vi "Init.vi"(8 "error in (no error)":errorcluster, 10 "Channel":i16, 11 "TrialBasedExperiment in":refnum<class "MouseMultiDim.lvclass">) -> (0 "error out":errorcluster, 3 "TrialBasedExperiment out":refnum<class "MouseMultiDim.lvclass">)   [LabVIEW 2014, in "MouseMultiDim.lvclass"]
uses:
  MouseMultiDim.lvclass
  Trial Based Experiment Statechart/PassiveExperiment/PassiveExperiment.lvclass
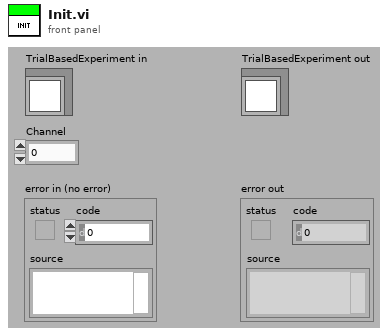
[diagram p1: front panel]
types:
  T1 = cluster{"Intertrial":dbl, "AcquireFixation":dbl, "HoldFixation":dbl, "DelayPeriod":dbl, "ResponsePeriod":dbl}
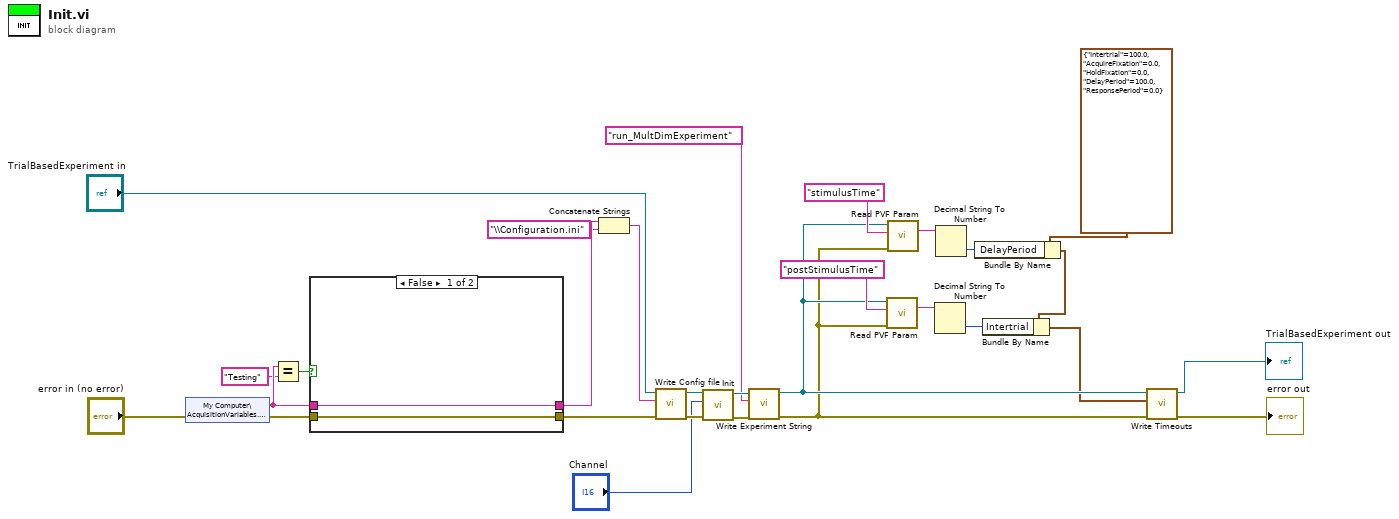
[diagram p0: block diagram]
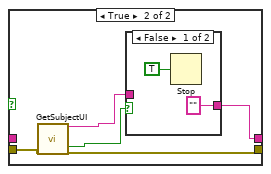
[diagram p2: hidden frame]
diagram:
  n1 = shared-variable "My Computer\\AcquisitionVariables.lvlib\\Subject"(error in="error in (no error)") -> (w26:string, error out=w27:errorcluster)
  n2 = Equal?(x=w26, y="Testing") -> (x = y?=w24:bool)
  n3 = case shown="False" w24 {
    tunnel: [w31 w36] -> w29
    tunnel: w26 -> [w31 _]
    tunnel: w27 -> [w30 w32]
    tunnel: [w30 w33] -> w28
    frame False {
    }
    frame True {
      n4 = call "GetSubjectUI.vi"("error in (no error)"=w32) -> ("subjectSelected"=w35:string, "OK"=w34:bool, "error out"=w33:errorcluster)  [unwired: 16 in]
      n5 = case shown="False" w34 {
        tunnel: w35 -> [_ w39]
        tunnel: ["" ("subjectSelected") w39] -> w36
        frame False {
          n6 = Stop(stop? (T)=TRUE) -> ()
        }
        frame True {
        }
      }
    }
  }
  n7 = Concatenate Strings(w29, "\\Configuration.ini") -> (w22:string)
  n8 = call-dynamic "Write Config file.vi"("error in (no error)"=w28, "Config file"=w22, "TrialBasedExperiment in"="TrialBasedExperiment in") -> ("error out"=w19:errorcluster, "TrialBasedExperiment out"=w21:refnum<class "MouseMultiDim.lvclass">)  [unwired: 7 in]
  n9 = call-parent "Init.vi"("error in (no error)"=w19, "Channel"="Channel", "TrialBasedExperiment in"=w21) -> ("error out"=w18:errorcluster, "TrialBasedExperiment out"=w20:refnum<class "MouseMultiDim.lvclass">)  [unwired: 7 in]
  n10 = call-dynamic "Write Experiment String.vi"("error in (no error)"=w18, "Experiment String"="run_MultDimExperiment" ("string"), "TrialBasedExperiment in"=w20) -> ("error out"=w3:errorcluster, "TrialBasedExperiment out"=w4:refnum<class "MouseMultiDim.lvclass">)  [unwired: 7 in]
  n11 = call-dynamic "Read PVF Param.vi"("error in (no error)"=w3, "Param Name"="postStimulusTime", "MatlabExperiment in"=w4) -> ("Param Value"=w6:string)  [unwired: 6 in, 2 out]
  n12 = call-dynamic "Read PVF Param.vi"("error in (no error)"=w3, "Param Name"="stimulusTime", "MatlabExperiment in"=w4) -> ("Param Value"=w9:string)  [unwired: 6 in, 2 out]
  n13 = Decimal String To Number(string=w6) -> (number=w5:i32)  [unwired: 2 in, 1 out]
  n14 = Decimal String To Number(string=w9) -> (number=w8:i32)  [unwired: 2 in, 1 out]
  n15 = Bundle By Name(cluster=T1 {"Intertrial"=100.0, "AcquireFixation"=0.0, "HoldFixation"=0.0, "DelayPeriod"=100.0, "ResponsePeriod"=0.0} ("Timeouts"), "DelayPeriod"=w8) -> (w2:T1)
  n16 = Bundle By Name(cluster=w2, "Intertrial"=w5) -> (w1:T1)
  n17 = call-dynamic "Write Timeouts.vi"("error in (no error)"=w3, "Timeouts"=w1, "TrialBasedExperiment in"=w4) -> ("error out"=→"error out":errorcluster, "TrialBasedExperiment out"=→"TrialBasedExperiment out":refnum<class "MouseMultiDim.lvclass">)  [unwired: 7 in]
